vi "Create XML Editor.vi"(5 "Common Doc Dir":string, 7 "CD Name":string, 8 "error in (no error)":errorcluster, 10 "XML Path":path) -> (0 "error out":errorcluster, 3 "Project XML Editor out":refnum<class "Project XML Editor.lvclass">)   [LabVIEW 2019, in "Project XML Editor.lvclass"]
uses:
  Project XML Editor.lvclass
  Project XML Editor.lvclass/Project XML Editor.ctl
  <vilib>/xml/Load XML File.vi
  <vilib>/xml/NI_XML.lvlib
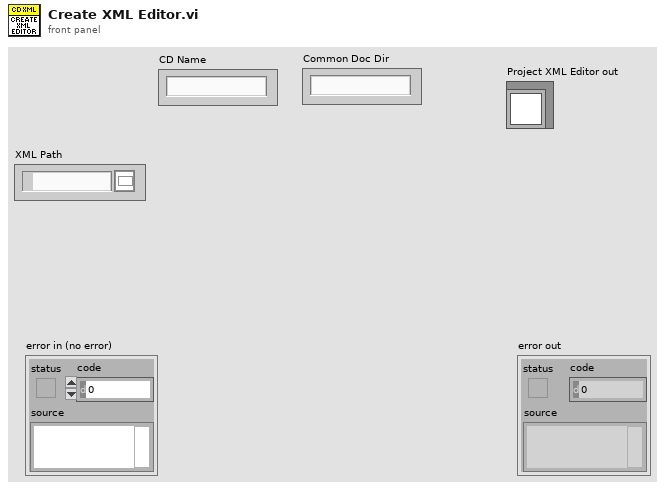
[diagram p1: front panel]
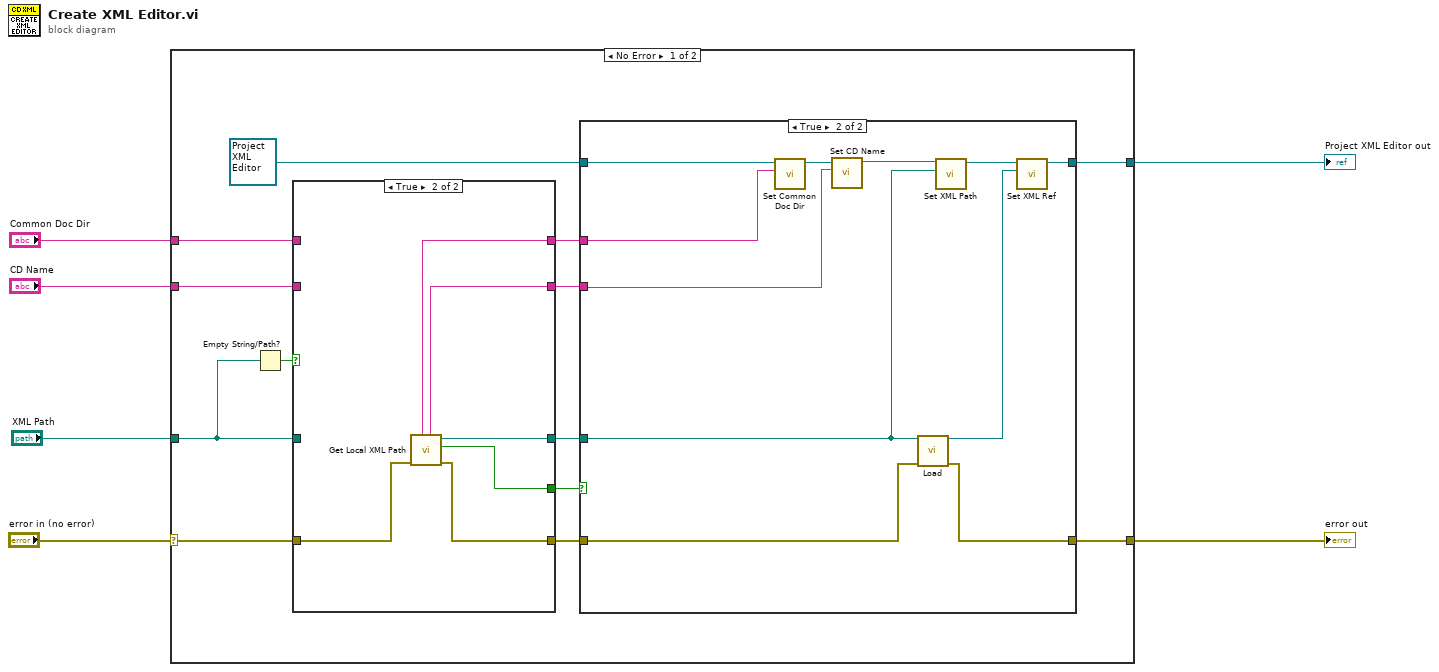
[diagram p0: block diagram]
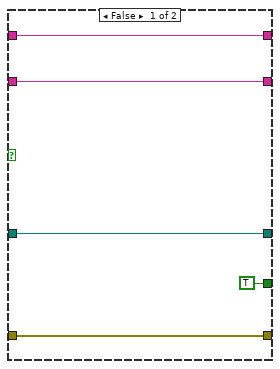
[diagram p3: hidden frame]
diagram:
  n1 = case shown="No Error" "error in (no error)" {
    selector: "error in (no error)" -> [w18 w44]
    tunnel: [w13 w44] -> w5
    tunnel: [w11 _] -> w4
    tunnel: "XML Path" -> [w17 _]
    tunnel: "Common Doc Dir" -> [w10 _]
    tunnel: "CD Name" -> [w9 _]
    frame No Error {
      n2 = Empty String/Path?(string/path=w17) -> (empty?=w19:bool)
      n3 = case shown="True" w19 {
        tunnel: w17 -> [w37 _]
        tunnel: w18 -> [w36 w43]
        tunnel: [w36 w42] -> w16
        tunnel: [w37 w41] -> w14
        tunnel: [TRUE ("Found ?") w40] -> w15
        tunnel: w10 -> [w34 _]
        tunnel: w9 -> [w33 _]
        tunnel: [w34 w39] -> w8
        tunnel: [w33 w38] -> w7
        frame False {
        }
        frame True {
          n4 = call "Get Local XML Path.vi"("Error In"=w43) -> ("Error Out"=w42:errorcluster, "Found ?"=w40:bool, "XML Path"=w41:path, "Custom Device Name"=w38:string, "Common Doc Dir"=w39:string)  [unwired: 6 in]
        }
      }
      n5 = case shown="True" w15 {
        tunnel: w16 -> [w21 w32]
        tunnel: w14 -> [_ w29]
        tunnel: [w21 w31] -> w13
        tunnel: refnum<class "Project XML Editor.lvclass"> refnum ("Project XML Editor in") -> [w20 w26]
        tunnel: [w20 w27] -> w11
        tunnel: w8 -> [_ w23]
        tunnel: w7 -> [_ w22]
        frame False {
        }
        frame True {
          n6 = call "Set Common Doc Dir.vi"("Common Doc Dir"=w23, "Project XML Editor in"=w26) -> ("Project XML Editor out"=w25:refnum<class "Project XML Editor.lvclass">)  [unwired: 9 in]
          n7 = call "Set CD Name.vi"("CD Name"=w22, "Project XML Editor in"=w25) -> ("Project XML Editor out"=w24:refnum<class "Project XML Editor.lvclass">)  [unwired: 9 in]
          n8 = call-poly <vilib>:"Load.vi"("path to XML document"=w29, "error in (no error)"=w32) -> ("DOM document out"=w28:refnum<k20>, "error out"=w31:errorcluster)  [unwired: 11 in, 1 out]
          n9 = call "Set XML Path.vi"("XML Path"=w29, "Project XML Editor in"=w24) -> ("Project XML Editor out"=w30:refnum<class "Project XML Editor.lvclass">)  [unwired: 9 in]
          n10 = call "Set XML Ref.vi"("XML Ref"=w28, "Project XML Editor in"=w30) -> ("Project XML Editor out"=w27:refnum<class "Project XML Editor.lvclass">)  [unwired: 9 in]
        }
      }
    }
    frame Error {
    }
  }
  "error out" <- w5
  "Project XML Editor out" <- w4
